vi "Set Neuron Properties.vi"(4 "Group":T1, 6 "Active":bool, 8 "Position Key":i32, 9 "InGROUP ID":i32, 10 "ID":i32, 11 "Neuron in":refnum<class "Neuron.lvclass">) -> (3 "Neuron out":refnum<class "Neuron.lvclass">)   [LabVIEW 2016, in "Neuron.lvclass"]
uses:
  Neuron.lvclass
  Controls/Type of Neuron.ctl
  Neuron.lvclass/Neuron.ctl
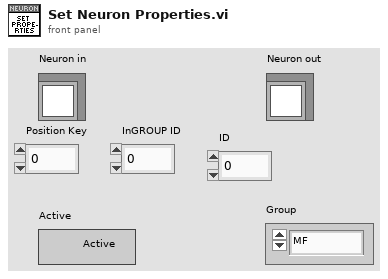
[diagram p1: front panel]
types:
  T1 = typedef "Type of Neuron.ctl" = enum16{"MF", "BA", "GO", "GC", "PC", "LU", "Glia (Dummy)"}
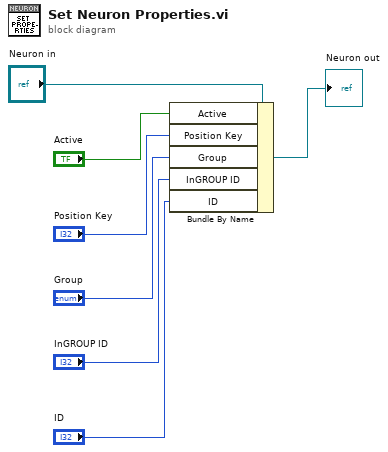
[diagram p0: block diagram]
diagram:
  n1 = Bundle By Name(cluster="Neuron in", "Active"="Active", "Position Key"="Position Key", "Group"="Group", "InGROUP ID"="InGROUP ID", "ID"="ID") -> (→"Neuron out":refnum<class "Neuron.lvclass">)
